vi "Set Enable State On Multiple Controls.vi"(8 "error in (no error)":errorcluster, 11 "Device in":refnum<class "Device.lvclass">) -> (0 "error out":errorcluster, 3 "Device out":refnum<class "Device.lvclass">)   [LabVIEW 2020, in "Device.lvlib" / "Device.lvclass"]
uses:
  Device.lvclass
panel:
  in  "Enable?":bool
  in  "Controls":refnum<vi>[](array[refnum])
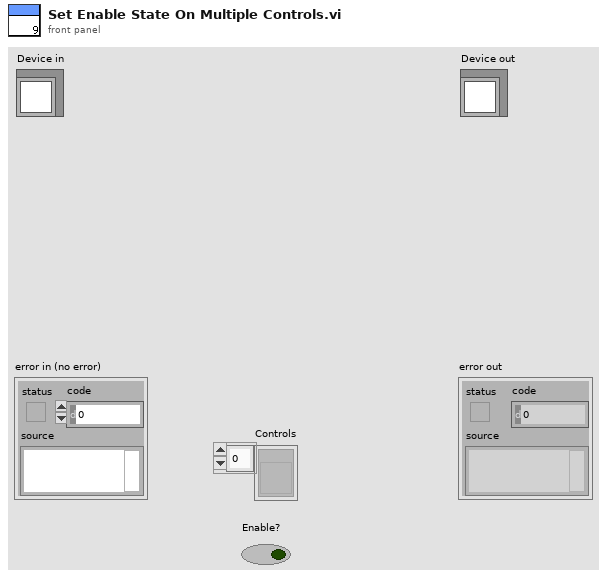
[diagram p1: front panel]
types:
  T1 = enum8{"Enabled", "Disabled", "Disabled and Grayed Out"}
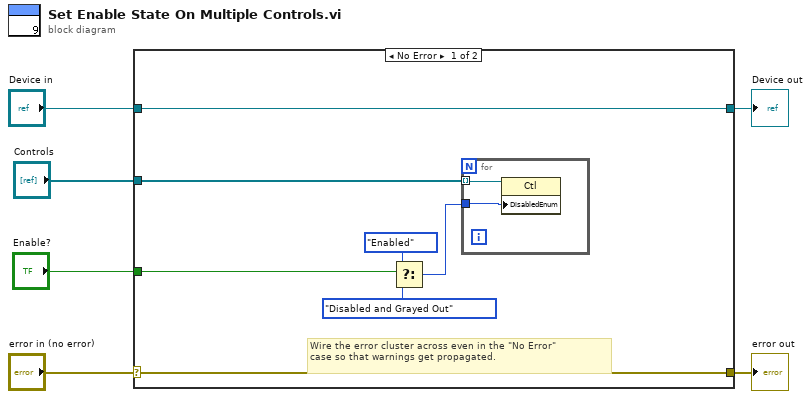
[diagram p0: block diagram]
diagram:
  n1 = case shown="No Error" "error in (no error)" {
    selector: "error in (no error)" -> [w12 w17]
    tunnel: [w12 w17] -> w5
    tunnel: [w13 w16] -> w3
    tunnel: "Device in" -> [w13 w16]
    tunnel: "Controls" -> [w8 _]
    tunnel: "Enable?" -> [w7 _]
    frame No Error {
      # "Wire the error cluster across even in the \"No Error\"\ncase so that warnings get propagated."
      n2 = Select(t=T1."Enabled" ("Disabled"), s=w7, f=T1."Disabled and Grayed Out" ("Disabled")) -> (s? t:f=w11:T1)
      n3 = for {
        tunnel: w8 -> [w15] mode=indexing
        tunnel: w11 -> [w14]
        n4 = property class="Ctl"(reference=w15, "DisabledEnum"=w14) -> ()  [unwired: 1 in, 2 out]
      }
    }
    frame Error {
    }
  }
  "error out" <- w5
  "Device out" <- w3
